vi "Read Voltage.vi"(8 "error in (no error)":errorcluster, 10 "Address (1)":u16=1 max=15 step=1, 11 "VISA resource name":refnum<visa-resource-name>) -> (0 "error out":errorcluster, 2 "Voltage (volts)":dbl, 3 "VISA resource name out":refnum<visa-resource-name>)   [LabVIEW 2021, in "Copy of Kloehn V6 Series.lvlib"]
doc: "Reads the instrument for the voltage. An 8-bit voltmeter is built into the pump I/O. It is accessible on pins 27 and 28 in the VersaPump 6 55 Series."
uses:
  Copy of Kloehn V6 Series.lvlib
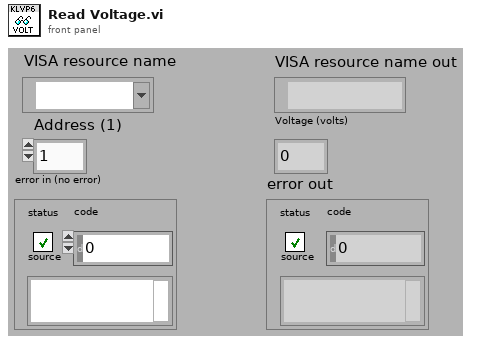
[diagram p1: front panel]
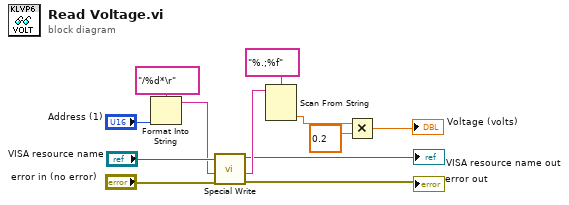
[diagram p0: block diagram]
diagram:
  n1 = Format Into String(format string="/%d*\r", "Address (1)") -> (resulting string=w2:string)  [unwired: 2 in, 1 out]
  n2 = call "Special Write.vi"("error in (no error)"="error in (no error)", "Send String"=w2, "VISA resource name"="VISA resource name") -> ("error out"=→"error out":errorcluster, "Parsed Response String"=w6:string, "VISA resource name out"=→"VISA resource name out":refnum<visa-resource-name>)  [unwired: 4 in, 2 out]
  n3 = Scan From String(format string="%.;%f", input string=w6) -> (output 1=w11:dbl)  [unwired: 3 in, 3 out]
  n4 = Multiply(x=w11, y=0.2) -> (x*y=→"Voltage (volts)":dbl)
